vi "parse_float32_roslv.vi"   [LabVIEW 2014]
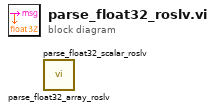
[diagram p0: block diagram]
diagram:
  n1 = call "parse_float32_array_roslv.vi"() -> ()  [unwired: 5 in, 3 out]
  n2 = call "parse_float32_scalar_roslv.vi"() -> ()  [unwired: 5 in, 3 out]
